vi "Tx Nested Content.vi"(8 "error in (no error)":errorcluster, 10 "Content":string, 11 "Root Actor in":refnum<class "Root Actor.lvclass">) -> (0 "error out":errorcluster, 3 "Root Actor out":refnum<class "Root Actor.lvclass">)   [LabVIEW 2020, in "Nested Actor.lvlib" / "Root Actor.lvclass"]
uses:
  Root Actor.lvclass
  Root Actor.lvclass/Root Actor.ctl
  Nested Actor Messages/Rcv Caller Content Msg/Rcv Caller Content Msg.lvclass/Rcv Caller Content Msg.ctl
  <vilib>/ActorFramework/Message Enqueuer/Message Enqueuer.lvclass/Message Enqueuer.ctl
  <vilib>/ActorFramework/Message Enqueuer/Enqueue.vi
  Nested Actor Messages/Rcv Caller Content Msg/Rcv Caller Content Msg.lvclass
  C:/Program Files (x86)/National Instruments/LabVIEW 2020/vi.lib/ActorFramework/Message/Message.lvclass
  <vilib>/ActorFramework/Message Priority Queue/Priority Enqueue.vi
  <vilib>/ActorFramework/Message Enqueuer/Message Enqueuer.lvclass
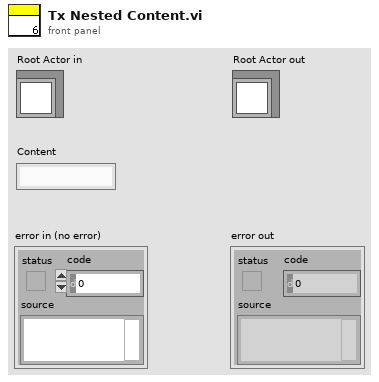
[diagram p1: front panel]
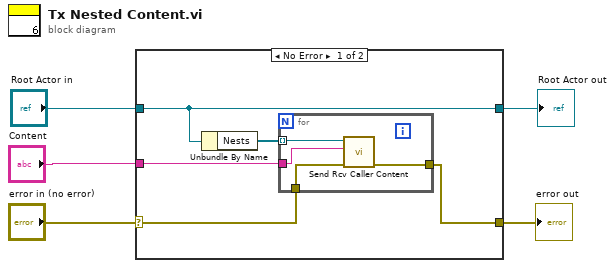
[diagram p0: block diagram]
diagram:
  n1 = case shown="No Error" "error in (no error)" {
    selector: "error in (no error)" -> [w7 w16]
    tunnel: [w6 w16] -> w4
    tunnel: [w10 w15] -> w2
    tunnel: "Root Actor in" -> [w10 w15]
    tunnel: "Content" -> [w8 _]
    frame No Error {
      n2 = Unbundle By Name(w10) -> ("Nests"=w9:refnum<class "Message Enqueuer.lvclass">[])
      n3 = for {
        tunnel: w9 -> [w14] mode=indexing
        tunnel: w8 -> [w13]
        tunnel: w7 -> [w12]
        tunnel: [w11] -> w6
        n4 = call "Send Rcv Caller Content.vi"("error in (no error)"=w12, "Content"=w13, "Message Enqueuer"=w14) -> ("error out"=w11:errorcluster)  [unwired: 7 in, 1 out]
      }
    }
    frame Error {
    }
  }
  "error out" <- w4
  "Root Actor out" <- w2
